vi "external trigger.vi"(7 "Daq parameters":T1={" Physical Channel"="PXI1Slot5/ai0:4", "Signal type"=10106, "Sample rate"=5000.0} {"Signal type" items=["default"=-1, "RSE"=10083, "NRSE"=10078, "Differential"=10106, "Pseudodifferential"=12529]}) -> ()   [LabVIEW 2012]
uses:
  <vilib>/DAQmx/read.llb/DAQmx Read (Analog 2D DBL NChan NSamp).vi
  <vilib>/DAQmx/create/channels.llb/DAQmx Create Channel (AI-Voltage-Basic).vi
  <vilib>/DAQmx/configure/timing.llb/DAQmx Timing (Sample Clock).vi
  <vilib>/DAQmx/configure/trigger.llb/DAQmx Start Trigger (Digital Edge).vi
  <vilib>/DAQmx/miscellaneous.llb/DAQmx Fill In Error Info.vi
panel:
  out "Waveform Graph":dbl[][](graph)
  in  "stop":bool
  in  "Trigger Source":tag="/PXI1Slot5/PFI0"
  # "Current Parameters"
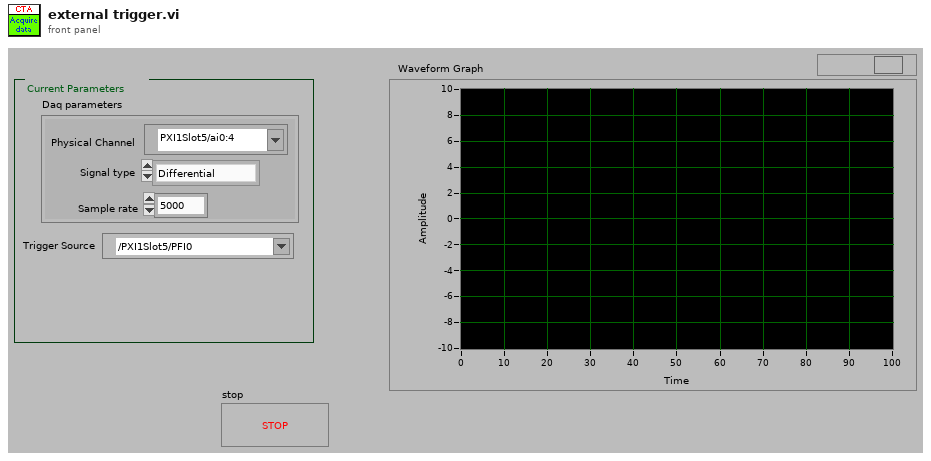
[diagram p1: front panel]
types:
  T1 = cluster{" Physical Channel":tag, "Signal type":i32, "Sample rate":dbl}
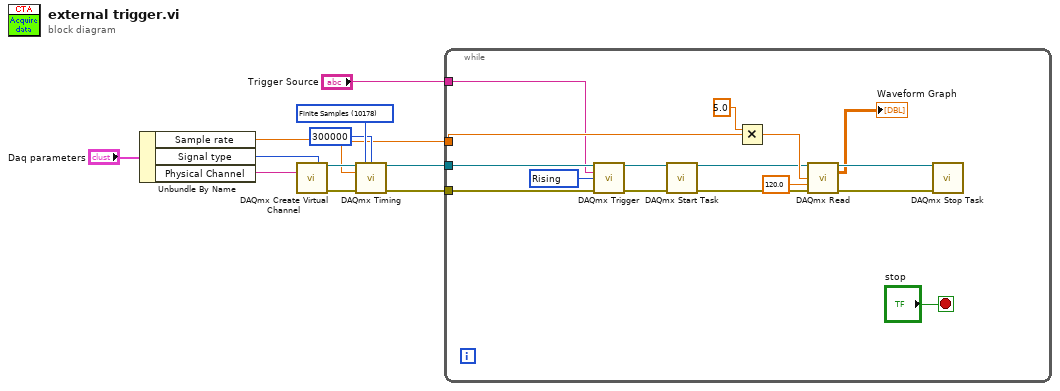
[diagram p0: block diagram]
diagram:
  w9 = 10178 items=["Finite Samples"=10178, "Continuous Samples"=10123, "Hardware Timed Single Point"=12522] ("sample mode")
  n1 = Unbundle By Name("Daq parameters") -> ("Sample rate"=w2:dbl, "Signal type"=w7:i32, "Physical Channel"=w8:tag)
  n2 = call-poly <vilib>:"DAQmx Create Virtual Channel.vi"("input terminal configuration"=w7, "physical channels"=w8) -> ("task out"=w11:refnum<k21>, "error out"=w10:errorcluster)  [unwired: 12 in]
  n3 = call-poly <vilib>:"DAQmx Timing.vi"("task/channels in"=w11, "sample mode"=w9, "samples per channel"=300000, "rate"=w2, "error in"=w10) -> ("task out"=w4:refnum<k21>, "error out"=w3:errorcluster)  [unwired: 9 in]
  n4 = while {
    tunnel: w3 -> [w25]
    tunnel: w4 -> [w26]
    tunnel: w2 -> [w27]
    tunnel: "Trigger Source" -> [w24]
    stop <- "stop" stop-if-true
    w21 = 10280 items=["Rising"=10280, "Falling"=10171] ("edge")
    n5 = call-poly <vilib>:"DAQmx Trigger.vi"("task/channels in"=w26, "source"=w24, "edge"=w21, "error in"=w25) -> ("task out"=w18:refnum<k21>, "error out"=w17:errorcluster)  [unwired: 10 in]
    n6 = call <vilib>:"DAQmx Start Task.vi"("task/channels in"=w18, "error in"=w17) -> ("task out"=w20:refnum<k21>, "error out"=w19:errorcluster)  [unwired: 12 in]
    n7 = Multiply(x=5.0, y=w27) -> (x*y=w23:dbl)
    n8 = call-poly <vilib>:"DAQmx Read.vi"("task/channels in"=w20, "number of samples per channel"=w23, "timeout"=120.0, "error in"=w19) -> ("task out"=w16:refnum<k21>, "data"=→"Waveform Graph":dbl[][], "error out"=w15:errorcluster)  [unwired: 9 in]
    n9 = call <vilib>:"DAQmx Stop Task.vi"("task/channels in"=w16, "error in"=w15) -> ()  [unwired: 12 in, 2 out]
  }
